vi "Kinect Shutdown Dani.vi"(8 "error in (no error)":errorcluster) -> (0 "error out":errorcluster)   [LabVIEW 2015]
uses:
  TypeDefs Host/Handle Enum.ctl
  libkinect_wrapper.dll
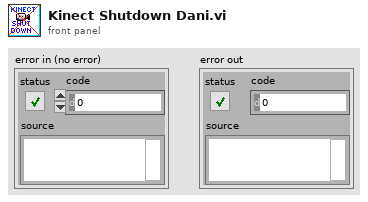
[diagram p1: front panel]
types:
  T1 = typedef "Handle Enum.ctl" = enum16{"Set Handles", "Get Handles"}
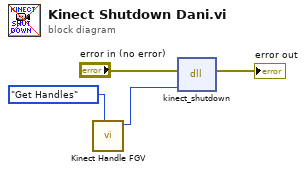
[diagram p0: block diagram]
diagram:
  n1 = call "Kinect Handle FGV.vi"("Handle Command"=Handle_Enum."Get Handles") -> ("Kinect Handle Out"=w1:i64)  [unwired: 9 in, 1 out]
  n2 = dll-call lib="libkinect_wrapper.*" fn="kinect_shutdown"(error in="error in (no error)", "Context_handle"=w1) -> (error out=→"error out":errorcluster)  [unwired: 4 in, 1 out]
